vi "字符串转换计算.vi"(10 "PC->PLC D寄存器":u16[](array[numeric]), 11 "读D寄存器长度":u16) -> (3 "字符串":string)   [LabVIEW 2014]
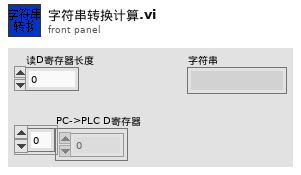
[diagram p1: front panel]
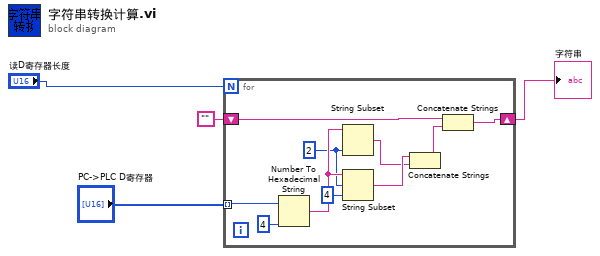
[diagram p0: block diagram]
diagram:
  n1 = for {
    N: "读D寄存器长度" -> [_]
    tunnel: "PC->PLC D寄存器" -> [w8] mode=indexing
    shift-right: [w5] -> w4
    shift-left: "" -> [w7]
    w12 = 2 ("长度（剩余）")
    n2 = Number To Hexadecimal String(1:i16 4 ("宽度(-)"), 2:w8) -> (0:w13:string)
    n3 = String Subset(string=w13, length (rest)=w12) -> (substring=w9:string)  [unwired: 1 in]
    n4 = String Subset(string=w13, offset (0)=w12, length (rest)=4 ("长度（剩余）")) -> (substring=w10:string)
    n5 = Concatenate Strings(w10, w9) -> (w6:string)
    n6 = Concatenate Strings(w7, w6) -> (w5:string)
  }
  "字符串" <- w4
